vi "TCP-IP Mgr.Create.vi"(6 "Working Dirs":T1, 7 "Ping Check":bool=TRUE, 8 "Error In":errorcluster, 11 "Q In":refnum<queue>) -> (0 "Error Out":errorcluster, 1 "Name Out":string, 3 "reference out":refnum<vi>)   [LabVIEW 2017, in "TCP-IP Mgr.lvlib"]
uses:
  TCP-IP Mgr.lvlib
  <vilib>/KATE/Queues/Q.Element.ctl
  <vilib>/KATE/Module/Module.Working Dirs.ctl
  <vilib>/KATE/Module/Module Utils.lvlib
  <vilib>/KATE/Queues/Queue Utils.lvlib
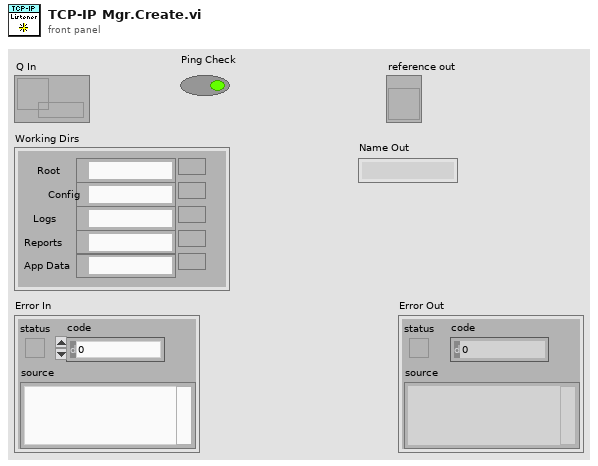
[diagram p1: front panel]
types:
  T1 = typedef "KATE_Lib.lvlib/Module Utils.lvlib/Module.Working Dirs.ctl" = cluster{"Root":path, "Config":path, "Logs":path, "Reports":path, "App Data":path}
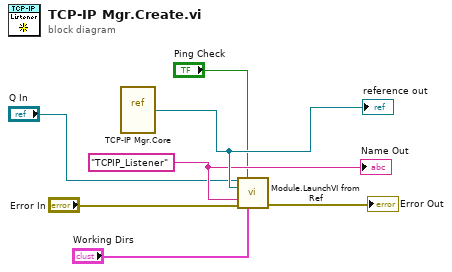
[diagram p0: block diagram]
diagram:
  w5 = "TCPIP_Listener" ("Name [Do not use!]")
  n1 = vi-ref "TCP-IP Mgr.Core.vi"() -> (w6:refnum<vi>)
  "reference out" <- w6
  n2 = call <vilib>:"Module.LaunchVI from Ref.vi"("Parent Q"="Q In", "Ping Check"="Ping Check", "VI Ref In"=w6, "Q Name"=w5, "error in"="Error In", "Working Dirs"="Working Dirs") -> ("error out"=→"Error Out":errorcluster)  [unwired: 7 in, 2 out]
  "Name Out" <- w5
